vi "HoppingStep(Nonlinear-XZ-SleepCtrl).vi"() -> ()   [LabVIEW 2014]
uses:
  <vilib>/Platform/TimedLoop/XDataNode/timing_clust.ctl
  <vilib>/Platform/TimedLoop/XDataNode/nitl_modes.ctl
  <vilib>/Platform/TimedLoop/XDataNode/wakeup.ctl
  <vilib>/rvi/Emulation/niFpgaGetClockAttributes.vi
  <vilib>/rvi/Emulation/niFpgaSctlEmulationGetInTimedLoop.vi
  <vilib>/rvi/Emulation/niFpgaEmulationReportErrorSimple.vi
  <vilib>/rvi/eio/common/nirviEmuTemplateMethod_errors.vi
  <vilib>/rvi/Emulation/niFpgaCriticalErrorInLSC.vi
  <vilib>/rvi/Emulation/niFpgaProcessEmulError.vi
  <vilib>/rvi/interface/RandomDataEmulation/niFpgaRandomDataHandleErrors.vi
  <vilib>/eio/EIONode/EIONode.xnode
  <vilib>/Platform/TimedLoop/XDataNode/XDataNode.xnode
  <vilib>/rvi/DataTransferAndStorage/Container/XNode/niFpgaContainer.xnode
  <vilib>/rvi/interface/RandomDataEmulation/nirviRandomDataFpgaReadWriteTemplate.vi
  <vilib>/Platform/TimedLoop/XDataNode/XDNodeRunTimeDep.lvlib
panel:
  in  "BottomSleep us":i16=80
  in  "UpperSleep us":i16=150
  in  "Relative?":bool
  out "ZRealPos":i16
  in  "RelativeWithdraw":i16
  out "Waveform Chart":i32(graph)
  in  "stop":bool
  out "Z":i32(graph)
  in  "ZOffset":i16
  in  "XOffset":i16
  in  "XNum":i16
  in  "XStepIndex":i16
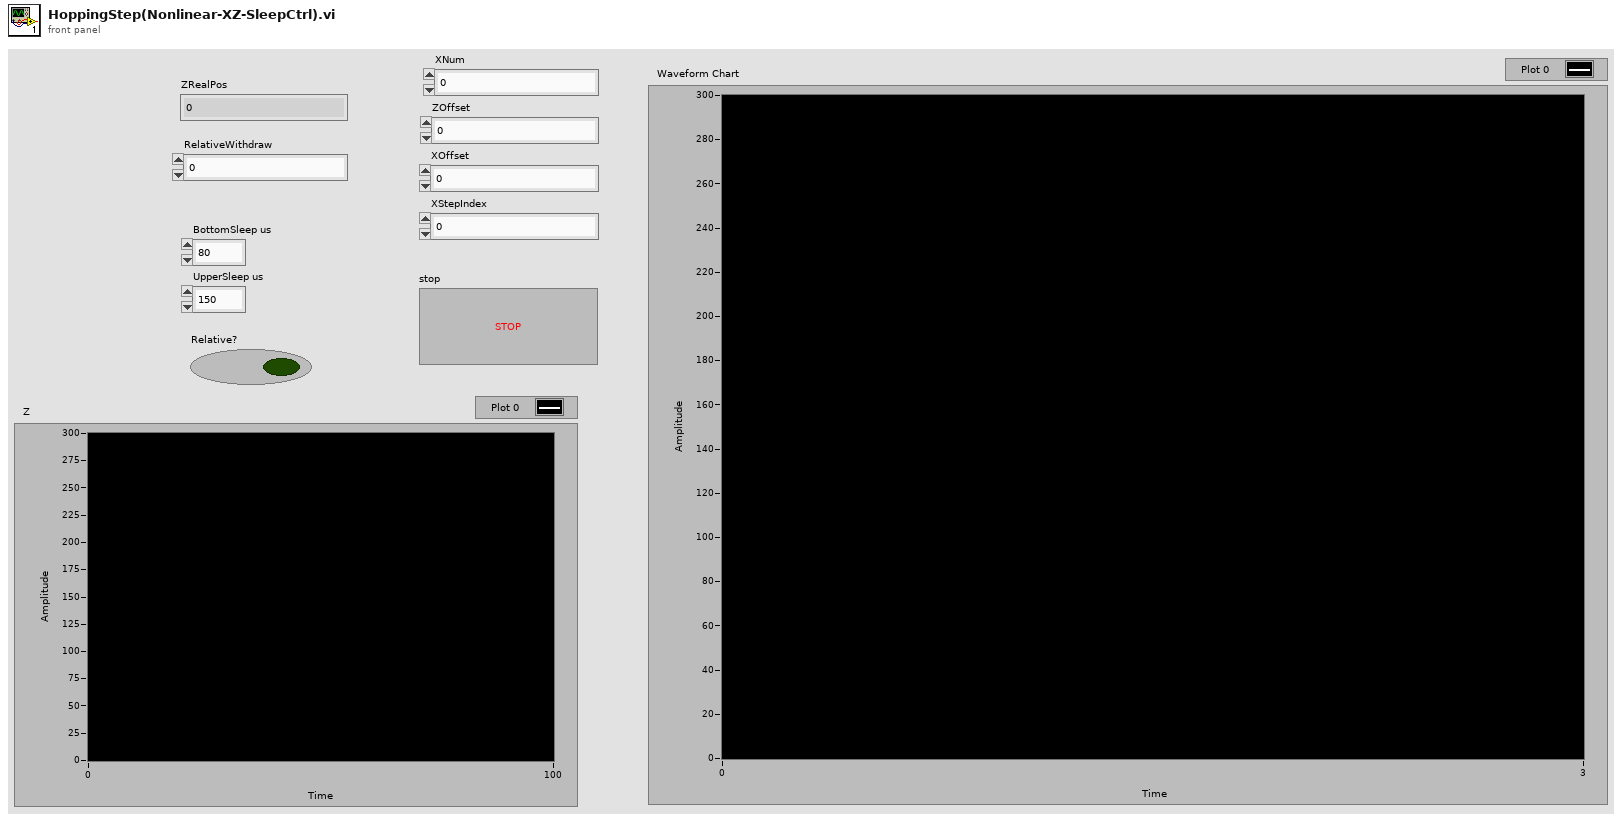
[diagram p1: front panel]
types:
  T1 = typedef "XDNodeRunTimeDep.lvlib/timing_clust.ctl" = cluster{"Expected End [f-1]":u64, "Actual End [f-1]":u64, "Finished Late? [f-1]":bool, "Expected End [i-1]":u64, "Actual End [i-1]":u64, "Finished Late? [i-1]":bool, "Expected Start [i]":u64, "Actual Start [i]":u64, "Expected Start [f]":u64, "Actual Start [f]":u64, "Source Name":string, "Structure Name":string, "Period":i64, "Deadline":i64, "Offset":i64, "Start":i64, "Priority":i32, "Timeout":i32, "Mode":T2, "Wakeup Reason":T3, "Error":errorcluster, "Source Type":string, "Secondary Source Type":string, "Global End Time":u64, "Global Start Time":u64, "Frame Duration":u64, "Iteration Duration":u64, "Assigned CPU":i32, "I/O Scan Engine Mode":u32}
  T2 = typedef "XDNodeRunTimeDep.lvlib/nitl_modes.ctl" = enum32{"No Change", "Process missed periods, maintain original phase", "Discard missed periods, maintain original phase", "Process missed periods, ignore original phase", "Discard missed periods, ignore original phase"}
  T3 = typedef "XDNodeRunTimeDep.lvlib/wakeup.ctl" = enum32{"Normal", "Aborted", "Asynchronous wakeup", "Timing source error", "Timed loop error", "Timeout"}
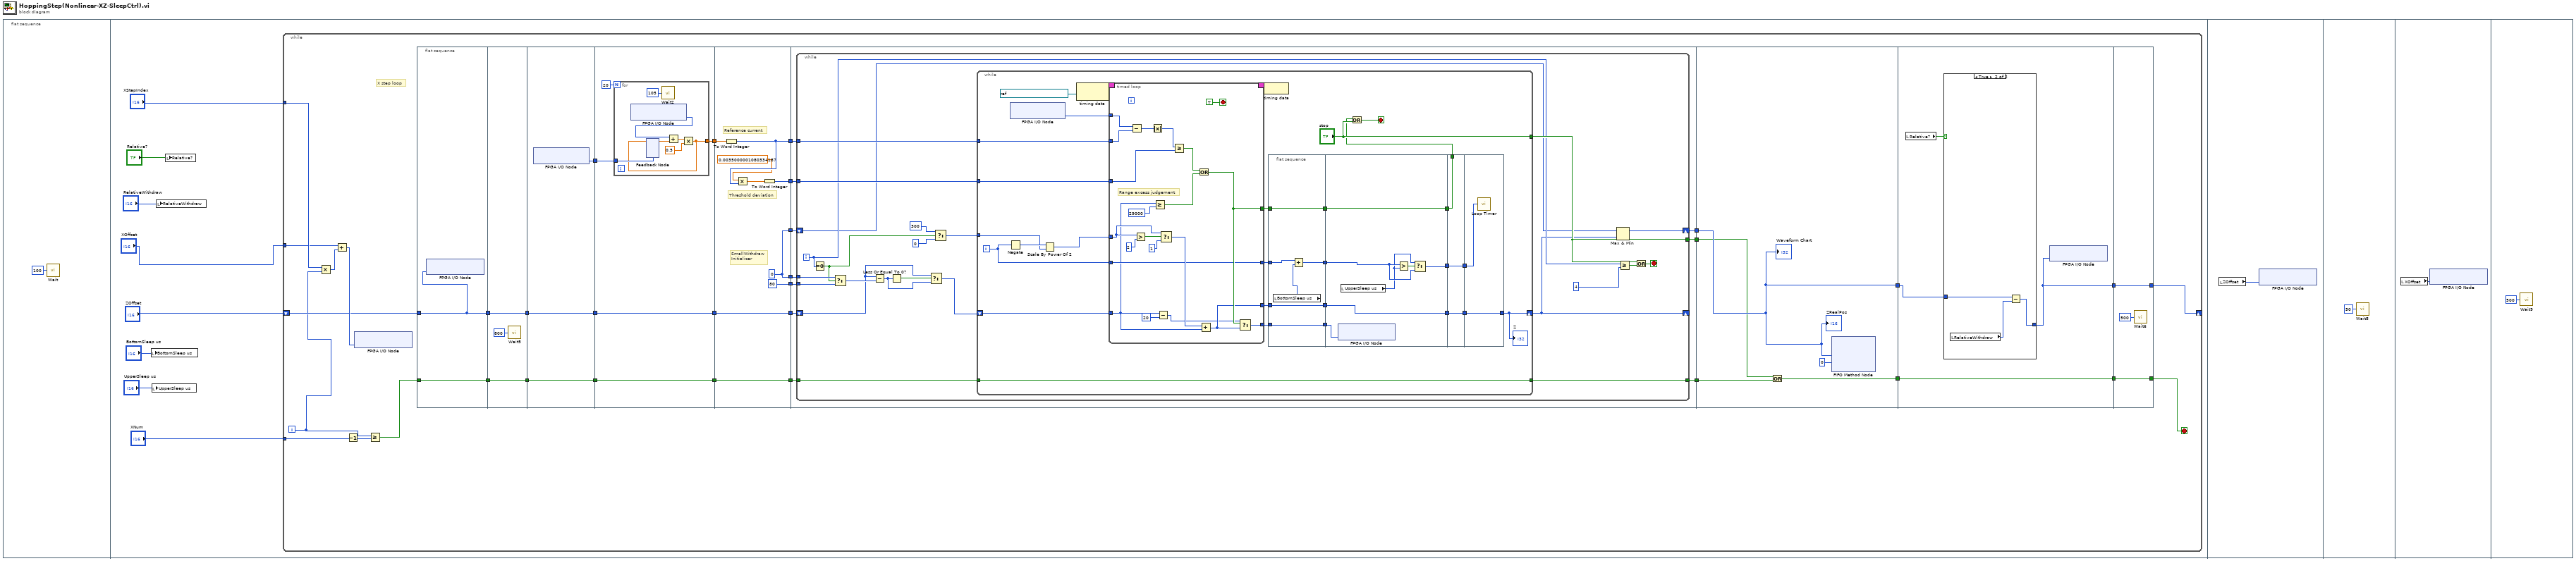
[diagram p0: block diagram]
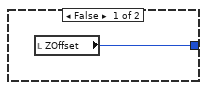
[diagram p2: hidden frame]
diagram:
  n1 = flat-sequence {
    frame #0 {
      n2 = call "Wait"("Count(mSec)"=u32 100 ("Count(uSec)")) -> ()  [unwired: 1 out]
    }
    frame #1 {
      n3 = local write "BottomSleep us"("BottomSleep us") -> ()
      n4 = local write "UpperSleep us"("UpperSleep us") -> ()
      n5 = local write "RelativeWithdraw"("RelativeWithdraw") -> ()
      n6 = local write "Relative?"("Relative?") -> ()
      n7 = while {
        tunnel: "XNum" -> [w29]
        tunnel: "XStepIndex" -> [w30]
        shift-right: [w19] -> _
        shift-left: "ZOffset" -> [w31]
        tunnel: "XOffset" -> [w22]
        i -> [w23]
        stop <- w39 stop-if-true
        # "X step loop"
        n8 = Multiply(x=w30, y=w23) -> (x*y=w35:i32)
        n9 = Add(x=w22, y=w35) -> (x+y=w36:i32)
        n10 = Decrement(x=w29) -> (x-1=w28:i16)
        n11 = xnode "FPGA I/O Node"("Connector0/AO2"=w36) -> ()  [unwired: 1 in, 1 out]
        n12 = Greater Or Equal?(x=w23, y=w28) -> (x >= y?=w27:bool)
        n13 = flat-sequence {
          tunnel: [w46] -> w13
          tunnel: w31 -> [w46]
          tunnel: w27 -> [w45]
          tunnel: [w45] -> w11
          tunnel: w13 -> [w49]
          tunnel: [w49] -> w12
          tunnel: w11 -> [w48]
          tunnel: [w48] -> w10
          tunnel: w12 -> [w52]
          tunnel: [w52] -> w16
          tunnel: w10 -> [w51]
          tunnel: [w51] -> w15
          tunnel: [w50] -> w14
          tunnel: [w56] -> w43
          tunnel: [w55] -> w37
          tunnel: w16 -> [w55]
          tunnel: w15 -> [w54]
          tunnel: [w54] -> w26
          tunnel: w14 -> [w53]
          tunnel: [w67] -> w44
          tunnel: w43 -> [w73]
          tunnel: [w72] -> w42
          tunnel: [w69] -> w41
          tunnel: [i16 80] -> w38
          tunnel: w37 -> [w67]
          tunnel: [w66] -> w34
          tunnel: [w66] -> w33
          tunnel: w26 -> [w65]
          tunnel: [w65] -> w25
          tunnel: w41 -> [w81]
          tunnel: w42 -> [w82]
          tunnel: w44 -> [w83]
          tunnel: [w80] -> w40
          tunnel: w38 -> [w79]
          tunnel: w34 -> [w78]
          tunnel: w33 -> [w77]
          tunnel: [w76] -> w32
          tunnel: w25 -> [w75]
          tunnel: [w74] -> w24
          tunnel: [w184] -> w21
          tunnel: [w183] -> w20
          tunnel: w24 -> [w181]
          tunnel: w32 -> [w183]
          tunnel: w40 -> [w182]
          tunnel: w21 -> [w189]
          tunnel: w20 -> [w188]
          tunnel: [w189] -> w18
          tunnel: [w187] -> w17
          tunnel: [w195] -> w19
          tunnel: [w196] -> w39
          tunnel: w18 -> [w196]
          tunnel: w17 -> [w195]
          frame #0 {
            n14 = xnode "FPGA I/O Node"("Connector0/AO0"=w46) -> ()  [unwired: 1 in, 1 out]
          }
          frame #1 {
            n15 = call "Wait5"("Count(uSec)"=u32 800) -> ()  [unwired: 1 out]
          }
          frame #2 {
            n16 = xnode "FPGA I/O Node"() -> ("Connector0/AI1"=w50:i16)  [unwired: 1 in, 1 out]
          }
          frame #3 {
            n17 = for {
              N: 20 -> [_]
              tunnel: [w58] -> w56
              tunnel: w53 -> [w60]
              n18 = xnode "FPGA I/O Node"() -> ("Connector0/AI1"=w59:i16)  [unwired: 1 in, 1 out]
              n19 = feedback #1(w60) -> (w63:sgl)
              n20 = call "Wait2"("Count(uSec)"=u32 105) -> ()  [unwired: 1 out]
              n21 = Add(x=w59, y=w63) -> (x+y=w62:sgl)
              n22 = Multiply(x=w62, y=sgl 0.5) -> (x*y=w58:sgl)
              n23 = feedback-in #1(w58) -> ()
            }
          }
          frame #4 {
            w66 = i16 0
            # "SmallWithdraw\nInitializer"
            # "Threshold deviation"
            # "Reference current"
            n24 = To Word Integer(number=w73) -> (16bit integer=w72:i16)
            n25 = Multiply(x=sgl 0.0035, y=w72) -> (x*y=w70:sgl)
            n26 = To Word Integer(number=w70) -> (16bit integer=w69:i16)
          }
          frame #5 {
            n27 = while {
              tunnel: w82 -> [w106]
              tunnel: w81 -> [w105]
              tunnel: [w102] -> w80
              tunnel: w79 -> [w100]
              shift-right: [w92] -> _
              shift-left: w83 -> [w97]
              tunnel: w78 -> [w94]
              shift-right: [w91] -> w76
              shift-left: w77 -> [w93]
              tunnel: w75 -> [w86]
              tunnel: [w85] -> w74
              i -> [w101]
              stop <- w104 stop-if-true
              n28 = Equal To 0?(x=w101) -> (x = 0?=w90:bool)
              n29 = Select(t=w94, s=w90, f=w100) -> (s? t:f=w99:i16)
              n30 = Subtract(x=w97, y=w99) -> (x-y=w96:i32)
              n31 = Less Or Equal To 0?(x=w96) -> (x <= 0?=w98:bool)
              n32 = Select(t=w97, s=w98, f=w96) -> (s? t:f=w95:i32)
              n33 = Select(t=i16 300, s=w90, f=i16 0) -> (s? t:f=w87:i16)
              n34 = while {
                tunnel: w106 -> [w128]
                tunnel: w105 -> [w130]
                tunnel: ["stop"] -> w102
                shift-right: [w120] -> w92
                shift-left: w95 -> [w125]
                tunnel: w87 -> [w110]
                tunnel: w86 -> [w107]
                tunnel: [w107] -> w85
                i -> [w108]
                stop <- w132 stop-if-true
                n35 = Negate(x=w108) -> (-x=w111:i32)
                n36 = xnode "FPGA I/O Node"() -> ("Connector0/AI1"=w129:i16)  [unwired: 1 in, 1 out]
                n37 = Scale By Power Of 2(n=w111, x=w110) -> (x*2^n=w109:i16)
                n38 = node-c288(refnum<k21> "40 MHz Onboard Clock" ("Source Name")) -> (w135:T1)
                n39 = timed-loop {
                  timing: w135 -> [_]
                  timing-out: [_] -> w134
                  tunnel: w128 -> [w172]
                  tunnel: w130 -> [w157]
                  tunnel: w129 -> [w173]
                  tunnel: [w168] -> w126
                  tunnel: [w167] -> w124
                  tunnel: w125 -> [w156]
                  tunnel: [w165] -> w122
                  tunnel: w109 -> [w160]
                  tunnel: [w162] -> w112
                  tunnel: w108 -> [w162]
                  stop <- TRUE stop-if-true
                  # "Range excess judgement"
                  n40 = Subtract(x=w173, y=w172) -> (x-y=w158:i16)
                  n41 = Greater?(x=w160, y=i16 2) -> (0:w159:bool)
                  n42 = Absolute Value(x=w158) -> (abs(x)=w171:i16)
                  n43 = Greater Or Equal?(x=w156, y=i16 29000) -> (x >= y?=w169:bool)
                  n44 = Subtract(x=w156, y=i16 20) -> (x-y=w154:i32)
                  n45 = Select(t=w160, s=w159, f=1) -> (s? t:f=w163:i32)
                  n46 = Greater Or Equal?(x=w171, y=w157) -> (x >= y?=w170:bool)
                  n47 = Or(x=w170, y=w169) -> (x .or. y?=w167:bool)
                  n48 = Add(x=w163, y=w156) -> (x+y=w165:i32)
                  n49 = Select(t=w154, s=w167, f=w165) -> (s? t:f=w168:i32)
                }
                n50 = node-c288(w134) -> ()
                n51 = flat-sequence {
                  tunnel: [w141] -> w127
                  tunnel: w126 -> [w141]
                  tunnel: w124 -> [w140]
                  tunnel: [w140] -> w123
                  tunnel: w122 -> [w139]
                  tunnel: [w139] -> w121
                  tunnel: [w137] -> w113
                  tunnel: w112 -> [w138]
                  tunnel: w127 -> [w146]
                  tunnel: [w148] -> w119
                  tunnel: w123 -> [w147]
                  tunnel: w121 -> [w148]
                  tunnel: [w147] -> w117
                  tunnel: [w144] -> w114
                  tunnel: w113 -> [w143]
                  tunnel: w119 -> [w151]
                  tunnel: [w151] -> w118
                  tunnel: w117 -> [w150]
                  tunnel: [w150] -> w116
                  tunnel: [w149] -> w115
                  tunnel: w114 -> [w149]
                  tunnel: w118 -> [w153]
                  tunnel: [w153] -> w120
                  tunnel: w115 -> [w152]
                  frame #0 {
                    n52 = local read "BottomSleep us"() -> (w136:i16)
                    n53 = Add(x=w138, y=w136) -> (x+y=w137:i32)
                  }
                  frame #1 {
                    n54 = xnode "FPGA I/O Node"("Connector0/AO0"=w146) -> ()  [unwired: 1 in, 1 out]
                    n55 = local read "UpperSleep us"() -> (w142:i16)
                    n56 = Greater?(x=w143, y=w142) -> (0:w145:bool)
                    n57 = Select(t=w142, s=w145, f=w143) -> (s? t:f=w144:i32)
                  }
                  frame #2 {
                  }
                  frame #3 {
                    n58 = call "Loop Timer"("Count(uSec)"=w152) -> ()  [unwired: 1 out]
                  }
                }
                n59 = Or(x=w116, y="stop") -> (x .or. y?=w132:bool)
                "Z" <- w120
              }
              n60 = Max & Min(x=w93, y=w92) -> (max(x,y)=w91:i32)  [unwired: 1 out]
              n61 = Greater Or Equal?(x=w101, y=4) -> (x >= y?=w103:bool)
              n62 = Or(x=w102, y=w103) -> (x .or. y?=w104:bool)
            }
          }
          frame #6 {
            n63 = Or(x=w182, y=w181) -> (x .or. y?=w184:bool)
            n64 = xnode ("FIFO Method Node")("Element"=w183, "Timeout"=0) -> ()  [unwired: 1 in, 2 out]
            "Waveform Chart" <- w183
            "ZRealPos" <- w183
          }
          frame #7 {
            n65 = local read "Relative?"() -> (w186:bool)
            n66 = case shown="True" w186 {
              tunnel: w188 -> [_ w193]
              tunnel: [w190 w191] -> w187
              frame False {
                n67 = local read "ZOffset"() -> (w190:i16)
              }
              frame True {
                n68 = local read "RelativeWithdraw"() -> (w192:i16)
                n69 = Subtract(x=w193, y=w192) -> (x-y=w191:i32)
              }
            }
            n70 = xnode "FPGA I/O Node"("Connector0/AO0"=w187) -> ()  [unwired: 1 in, 1 out]
          }
          frame #8 {
            n71 = call "Wait6"("Count(uSec)"=u32 500) -> ()  [unwired: 1 out]
          }
        }
      }
    }
    frame #2 {
      n72 = local read "ZOffset"() -> (w197:i16)
      n73 = xnode "FPGA I/O Node"("Connector0/AO0"=w197) -> ()  [unwired: 1 in, 1 out]
    }
    frame #3 {
      n74 = call "Wait8"("Count(uSec)"=u32 50) -> ()  [unwired: 1 out]
    }
    frame #4 {
      n75 = local read "XOffset"() -> (w199:i16)
      n76 = xnode "FPGA I/O Node"("Connector0/AO2"=w199) -> ()  [unwired: 1 in, 1 out]
    }
    frame #5 {
      n77 = call "Wait9"("Count(uSec)"=u32 500) -> ()  [unwired: 1 out]
    }
  }
